vi "compare-trapezoid-profile-position-ctrl.vi"() -> ()   [LabVIEW 2019]
uses:
  Secret_Control_Library_Protected/CtrlTrain_Pos_ctrl_TuningParameters.ctl
  <vilib>/Rock Robotics/WPI/ThirdParty/JAS_Junk/TrajLib/SlewRateLimiter_New.vi
  <vilib>/Rock Robotics/WPI/ThirdParty/JAS_Junk/TrajLib/SlewRateLimiter_Reset.vi
  <vilib>/Rock Robotics/WPI/ThirdParty/JAS_Junk/TrajLib/SlewRateLimiter_Calculate.vi
  <vilib>/Rock Robotics/WPI/ThirdParty/JAS_Junk/TrajLib/SlewRateLimiter_SetRate.vi
  <vilib>/Rock Robotics/WPI/ThirdParty/JAS_Junk/TrajLib/TrapProfile_Calculate.vi
  <vilib>/Rock Robotics/WPI/ThirdParty/JAS_Junk/TrajLib/TrapProfile_New.vi
  <vilib>/Rock Robotics/WPI/ThirdParty/JAS_Junk/TrajLib/TrapProfile_TotalTime.vi
  <vilib>/Rock Robotics/WPI/ThirdParty/JAS_Junk/TrajLib/TrapProfConstraint_New.vi
  <vilib>/Rock Robotics/WPI/ThirdParty/JAS_Junk/TrajLib/TrapProfState_New.vi
  <vilib>/Rock Robotics/WPI/ThirdParty/JAS_Junk/TrajLib/TrapProfile_IsFinished.vi
  <vilib>/Rock Robotics/WPI/ThirdParty/JAS_Junk/TrajLib/TrapProfile_Direct.vi
  <vilib>/Rock Robotics/WPI/ThirdParty/JAS_Junk/TrajLib/TrapProfile_ShouldFlipAcceleration.vi
  <vilib>/Rock Robotics/SystemInterfaces/NetworkCommunication/NetComm_UsageReport_report.vi
  <vilib>/addons/control/pid/pid.llb/PID Lead-Lag (DBL).vi
  <vilib>/Rock Robotics/WPI/ThirdParty/JAS_Junk/TrajLib/Util_LibraryGlobals.vi
  <vilib>/Rock Robotics/WPI/ThirdParty/JAS_Junk/TrajLib/Util_GetTime.vi
  <vilib>/addons/control/pid/NI_PID_pid.lvlib
  <vilib>/Rock Robotics/WPI/ThirdParty/JAS_Junk/TrajLib/Trajectory_Library.lvlib
  Secret_Control_Library_Protected/Secret_Control_Library_Protected.lvlib
panel:
  in  "Tab Control":T1(tab)
  out "PC-SP, PV, CO Chart":T2(graph)
  in  "Desired Position":dbl(slide) min=0.0 max=90.0 scale=0.0..90.0
  in  "Auto - Set Position To 0 / Manual - Lower":bool
  in  "Auto - Set Position to 90 / Manual - Raise":bool
  in  "Set Position to Desired\n(Select to activate position)":bool
  out "Selected Setpoint \n(In Manual \ntracks Position)":dbl
  out "Trap-Current \nPosition 2":dbl format="%.2f"
  out "Trap-Motor \nDemand2":dbl format="%#.2f"
  out "Trap-Position Error":dbl format="%#3.2f"
  out "Trap-SP, PV, CO Chart":T2(graph)
  out "Trap-Current Position":dbl(knob) scale=-10.0..100.0
  in  "Auto / Manual":bool=TRUE
  in  "MinLimitSwitch":bool
  in  "MaxLimitSwitch":bool
  out "Trap-In Position":bool
  out "PC-Current \nPosition 2":dbl format="%.2f"
  out "PC-Motor \nDemand 2":dbl format="%#.2f"
  out "PC-Current Position 3":dbl(knob) scale=-10.0..100.0
  out "Selected Setpoint \n(In Manual \ntracks Position) 2":dbl
  out "PC-In Position":bool
  out "PC-Position Error":dbl format="%#3.2f"
  in  "MaxLimitSwitch 2":bool
  in  "MinLimitSwitch 2":bool
  in  "Trap-Max Accel":dbl=10.6 format="%#_13g"
  in  "PC-TuningParameters":T3={"MaxOutput"=1.0, "MinOutput"=0.25, "PositionErrThreshold"=6.0, "PositionErrDeadband"=0.5, "ReverseOutput"=FALSE, "PositionMax"=89.0, "PositionMin"=1.0, "WithinDBCount"=5} {"WithinDBCount" min=1}
  in  "trap-PositionTolerance":dbl=0.5 format="%#_13g"
  in  "Trap-VelocityTolerance":dbl=1.0 format="%#_13g"
  in  "Trap-ConsecutiveAtGoalCount":i32=5
  in  "Trap-Max Speed":dbl=8.5 format="%#_13g"
  in  "PC-MaxAccelRate":dbl=1.25 format="%#_13g"
  out "Both-Current-Setpoint":dbl
  out "Trap-Current-Position":dbl
  out "Both-Manual-Lower":bool
  out "Both-Manual-Raise":bool
  out "Trap-Motor-Demand":dbl
  out "PC-Current-Position":dbl
  out "PC-Motor-Demand":dbl
  # "Compare trapezoid with position control"
  # "Toggle these switches to simulate a limit switch input."
  # "Max Vel = 8.5"
  # "Max Output = 1.0"
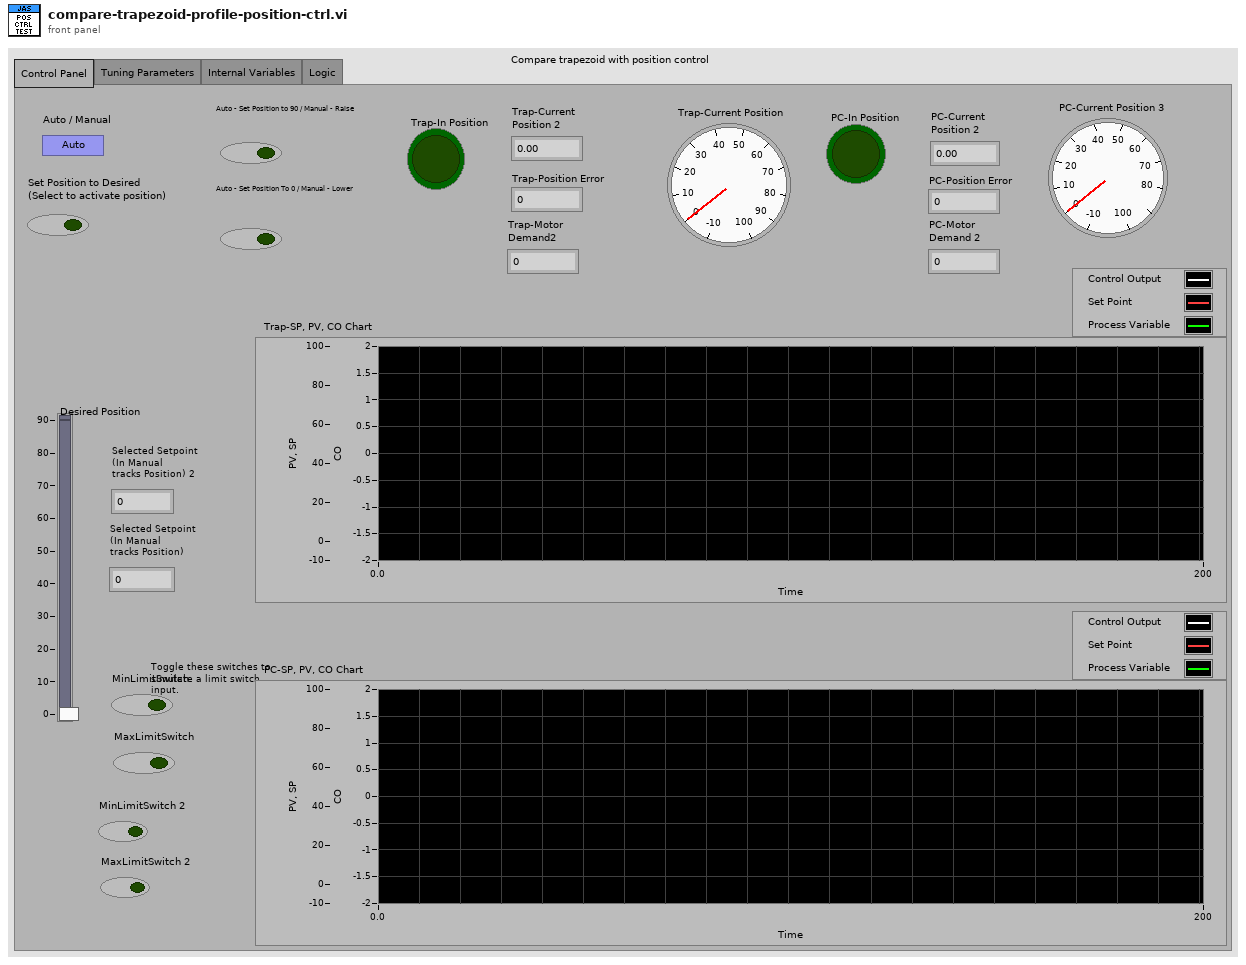
[diagram p1: front panel]
types:
  T1 = enum32{"Control Panel", "Tuning Parameters", "Internal Variables", "Logic"}
  T2 = cluster{"MotorDemand":dbl, "CurrentSetpoint":dbl, "CurrentPosition":dbl}
  T3 = typedef "Secret_Control_Library_Protected.lvlib/CtrlTrain_Pos_ctrl_TuningParameters.ctl" = cluster{"MaxOutput":dbl, "MinOutput":dbl, "PositionErrThreshold":dbl, "PositionErrDeadband":dbl, "ReverseOutput":bool, "PositionMax":dbl, "PositionMin":dbl, "WithinDBCount":i32}
  T4 = cluster{"gain":dbl, "lag time":dbl, "lead time":dbl}
  T5 = cluster{"PC-Motor-Demand":dbl, "Both-Current-Setpoint":dbl, "PC-Current-Position":dbl}
  T6 = cluster{"Trap-Motor-Demand":dbl, "Both-Current-Setpoint":dbl, "Trap-Current-Position":dbl}
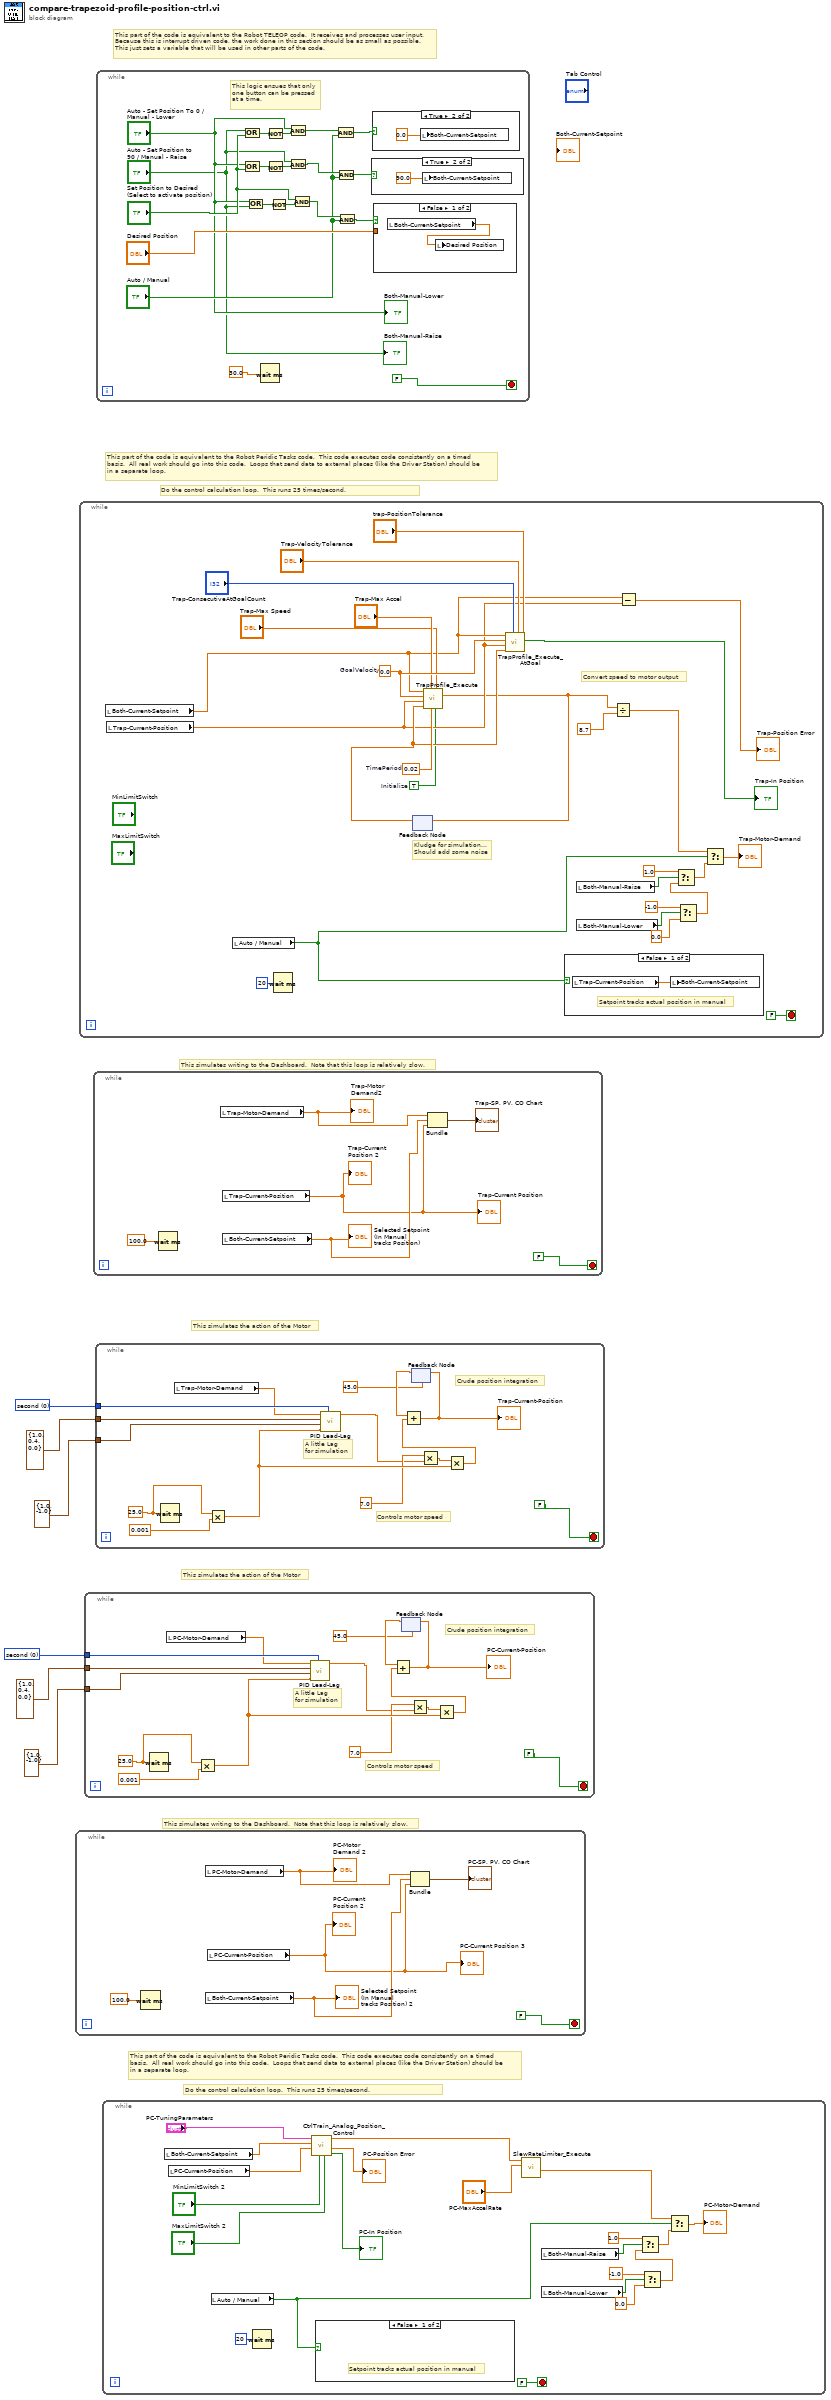
[diagram p0: block diagram]
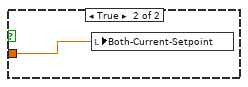
[diagram p4: hidden frame]
diagram:
  w1 = u16 0 items=["second", "minute"] ("time unit")
  w6 = u16 0 items=["second", "minute"] ("time unit")
  # "Do the control calculation loop.  This runs 25 times/second."
  # "This part of the code is equivalent to the Robot Peridic Tasks code.  This code executes code consistently on a timed\nbasis.  All real work should go into this code.  Loops that send data to external places (like the Driver Station) should be \nin a separate loop."
  # "This simulates writing to the Dashboard.  Note that this loop is relatively slow."
  # "This simulates the action of the Motor"
  # "This simulates the action of the Motor"
  # "This simulates writing to the Dashboard.  Note that this loop is relatively slow."
  # "Do the control calculation loop.  This runs 25 times/second."
  # "This part of the code is equivalent to the Robot Peridic Tasks code.  This code executes code consistently on a timed\nbasis.  All real work should go into this code.  Loops that send data to external places (like the Driver Station) should be \nin a separate loop."
  # "This part of the code is equivalent to the Robot TELEOP code.  It receives and processes user input.\nBecause this is interrupt driven code, the work done in this section should be as small as possible.\nThis just sets a variable that will be used in other parts of the code."
  n1 = while {
    stop <- FALSE stop-if-true
    n2 = Wait (ms)(milliseconds to wait=100.0) -> ()  [unwired: 1 out]
    n3 = local read "PC-Motor-Demand"() -> (w8:dbl)
    "PC-Motor \nDemand 2" <- w8
    n4 = local read "Both-Current-Setpoint"() -> (w10:dbl)
    "Selected Setpoint \n(In Manual \ntracks Position) 2" <- w10
    n5 = local read "PC-Current-Position"() -> (w9:dbl)
    "PC-Current \nPosition 2" <- w9
    "PC-Current Position 3" <- w9
    n6 = Bundle("PC-Motor-Demand"=w8, "Both-Current-Setpoint"=w10, "PC-Current-Position"=w9) -> (→"PC-SP, PV, CO Chart":T5)  [unwired: 1 in]
  }
  n7 = while {
    stop <- FALSE stop-if-true
    w29 = 0.0  # GoalVelocity
    w24 = 0.02  # TimePeriod
    w13 = TRUE  # Initialize
    # "Convert speed to motor output"
    # "Kludge for simulation...\nShould add some noise"
    n8 = local read "Both-Current-Setpoint"() -> (w21:dbl)
    n9 = local read "Trap-Current-Position"() -> (w17:dbl)
    n10 = local read "Auto / Manual"() -> (w34:bool)
    n11 = Wait (ms)(milliseconds to wait=u32 20) -> ()  [unwired: 1 out]
    n12 = feedback #1() -> (w18:dbl)  [unwired: 1 in]
    n13 = call <vilib>:"TrapProfile_Execute.vi"("Initialize"=w13, "Max Speed"="Trap-Max Speed", "TimePeriod"=w24, "Max Accel"="Trap-Max Accel", "CurrentVelocity"=w18, "CurrentPosition"=w17, "GoalVelocity"=w29, "GoalPosition"=w21) -> ("VelocityDmd"=w14:dbl)  [unwired: 3 out]
    n14 = feedback-in #1(w14) -> ()
    n15 = call <vilib>:"TrapProfile_Execute_AtGoal.vi"("PositionTolerance"="trap-PositionTolerance", "VelocityTolerance"="Trap-VelocityTolerance", "ConsecutiveAtGoalCount"="Trap-ConsecutiveAtGoalCount", "CurrentVelocity"=w18, "CurrentPosition"=w17, "GoalVelocity"=w29, "GoalPosition"=w21) -> ("AtGoal"=→"Trap-In Position":bool)  [unwired: 4 in]
    n16 = case shown="False" w34 {
      frame False {
        # "Setpoint tracks actual position in manual"
        n17 = local read "Trap-Current-Position"() -> (w40:dbl)
        n18 = local write "Both-Current-Setpoint"(w40) -> ()
      }
      frame True {
      }
    }
    n19 = local read "Both-Manual-Raise"() -> (w33:bool)
    n20 = local read "Both-Manual-Lower"() -> (w32:bool)
    n21 = Divide(x=w14, y=8.7) -> (x/y=w15:dbl)
    n22 = Subtract(x=w21, y=w17) -> (x-y=→"Trap-Position Error":dbl)
    n23 = Select(t=-1.0, s=w32, f=0.0) -> (s? t:f=w36:dbl)
    n24 = Select(t=1.0, s=w33, f=w36) -> (s? t:f=w35:dbl)
    n25 = Select(t=w15, s=w34, f=w35) -> (s? t:f=→"Trap-Motor-Demand":dbl)
  }
  n26 = while {
    tunnel: w1 -> [w55]
    tunnel: T4 {"gain"=1.0, "lag time"=0.4, "lead time"=0.0} ("tuning parameters") -> [w54]
    tunnel: cluster{"output high":dbl, "output low":dbl} {"output high"=1.0, "output low"=-1.0} ("output range") -> [w52]
    stop <- FALSE stop-if-true
    w44 = 25.0
    # "Controls motor speed"
    # "Crude position integration"
    # "A little Lag\nfor simulation"
    n27 = Wait (ms)(milliseconds to wait=w44) -> ()  [unwired: 1 out]
    n28 = local read "PC-Motor-Demand"() -> (w41:dbl)
    n29 = Multiply(x=w44, y=0.001) -> (x*y=w51:dbl)
    n30 = call-poly <vilib>:"PID Lead-Lag.vi"("time unit"=w55, "dt (s)"=w51, "output range"=w52, "tuning parameters"=w54, "input"=w41) -> ("output"=w43:dbl)  [unwired: 3 in, 1 out]
    n31 = feedback #2(45.0) -> (w49:dbl)
    n32 = Multiply(x=7.0, y=w43) -> (x*y=w50:dbl)
    n33 = Multiply(x=w50, y=w51) -> (x*y=w47:dbl)
    n34 = Add(x=w49, y=w47) -> (x+y=w42:dbl)
    "PC-Current-Position" <- w42
    n35 = feedback-in #2(w42) -> ()
  }
  n36 = while {
    stop <- FALSE stop-if-true
    n37 = Wait (ms)(milliseconds to wait=100.0) -> ()  [unwired: 1 out]
    n38 = local read "Trap-Motor-Demand"() -> (w56:dbl)
    "Trap-Motor \nDemand2" <- w56
    n39 = local read "Trap-Current-Position"() -> (w57:dbl)
    "Trap-Current \nPosition 2" <- w57
    "Trap-Current Position" <- w57
    n40 = local read "Both-Current-Setpoint"() -> (w58:dbl)
    "Selected Setpoint \n(In Manual \ntracks Position)" <- w58
    n41 = Bundle("Trap-Motor-Demand"=w56, "Both-Current-Setpoint"=w58, "Trap-Current-Position"=w57) -> (→"Trap-SP, PV, CO Chart":T6)  [unwired: 1 in]
  }
  n42 = while {
    tunnel: w6 -> [w76]
    tunnel: T4 {"gain"=1.0, "lag time"=0.4, "lead time"=0.0} ("tuning parameters") -> [w75]
    tunnel: cluster{"output high":dbl, "output low":dbl} {"output high"=1.0, "output low"=-1.0} ("output range") -> [w73]
    stop <- FALSE stop-if-true
    w65 = 25.0
    # "Controls motor speed"
    # "Crude position integration"
    # "A little Lag\nfor simulation"
    n43 = Wait (ms)(milliseconds to wait=w65) -> ()  [unwired: 1 out]
    n44 = local read "Trap-Motor-Demand"() -> (w62:dbl)
    n45 = Multiply(x=w65, y=0.001) -> (x*y=w72:dbl)
    n46 = call-poly <vilib>:"PID Lead-Lag.vi"("time unit"=w76, "dt (s)"=w72, "output range"=w73, "tuning parameters"=w75, "input"=w62) -> ("output"=w64:dbl)  [unwired: 3 in, 1 out]
    n47 = feedback #3(45.0) -> (w70:dbl)
    n48 = Multiply(x=7.0, y=w64) -> (x*y=w71:dbl)
    n49 = Multiply(x=w71, y=w72) -> (x*y=w68:dbl)
    n50 = Add(x=w70, y=w68) -> (x+y=w63:dbl)
    "Trap-Current-Position" <- w63
    n51 = feedback-in #3(w63) -> ()
  }
  n52 = while {
    stop <- FALSE stop-if-true
    # "This logic ensues that only\none button can be pressed\nat a time."
    n53 = Or(x="Auto - Set Position to 90 / Manual - Raise", y="Set Position to Desired\n(Select to activate position)") -> (x .or. y?=w95:bool)
    n54 = Or(x="Auto - Set Position To 0 / Manual - Lower", y="Set Position to Desired\n(Select to activate position)") -> (x .or. y?=w93:bool)
    n55 = Or(x="Auto - Set Position To 0 / Manual - Lower", y="Auto - Set Position to 90 / Manual - Raise") -> (x .or. y?=w91:bool)
    n56 = Wait (ms)(milliseconds to wait=30.0) -> ()  [unwired: 1 out]
    n57 = Not(x=w95) -> (.not. x?=w94:bool)
    n58 = Not(x=w93) -> (.not. x?=w92:bool)
    n59 = Not(x=w91) -> (.not. x?=w90:bool)
    n60 = And(x="Auto - Set Position To 0 / Manual - Lower", y=w94) -> (x .and. y?=w85:bool)
    n61 = And(x="Auto - Set Position to 90 / Manual - Raise", y=w92) -> (x .and. y?=w81:bool)
    n62 = And(x="Set Position to Desired\n(Select to activate position)", y=w90) -> (x .and. y?=w80:bool)
    n63 = And(x=w85, y="Auto / Manual") -> (x .and. y?=w84:bool)
    n64 = And(x=w81, y="Auto / Manual") -> (x .and. y?=w83:bool)
    n65 = And(x=w80, y="Auto / Manual") -> (x .and. y?=w82:bool)
    n66 = case shown="True" w83 {
      frame False {
      }
      frame True {
        n67 = local write "Both-Current-Setpoint"(90.0) -> ()
      }
    }
    n68 = case shown="True" w84 {
      frame False {
      }
      frame True {
        n69 = local write "Both-Current-Setpoint"(0.0) -> ()
      }
    }
    n70 = case shown="False" w82 {
      tunnel: "Desired Position" -> [_ w97]
      frame False {
        n71 = local read "Both-Current-Setpoint"() -> (w96:dbl)
        n72 = local write "Desired Position"(w96) -> ()
      }
      frame True {
        n73 = local write "Both-Current-Setpoint"(w97) -> ()
      }
    }
    "Both-Manual-Raise" <- "Auto - Set Position to 90 / Manual - Raise"
    "Both-Manual-Lower" <- "Auto - Set Position To 0 / Manual - Lower"
  }
  n74 = while {
    stop <- FALSE stop-if-true
    n75 = local read "Both-Current-Setpoint"() -> (w109:dbl)
    n76 = local read "PC-Current-Position"() -> (w108:dbl)
    n77 = local read "Auto / Manual"() -> (w115:bool)
    n78 = Wait (ms)(milliseconds to wait=u32 20) -> ()  [unwired: 1 out]
    n79 = call "CtrlTrain_Analog_Position_Control.vi"("PositionMax"="MaxLimitSwitch 2", "PositionMin"="MinLimitSwitch 2", "CurrentPosition"=w108, "TargetPosition"=w109, "Pos_Ctrl_TuningParameters"="PC-TuningParameters") -> ("OnTarget"=→"PC-In Position":bool, "PositionError"=→"PC-Position Error":dbl, "Output"=w101:dbl)  [unwired: 4 in]
    n80 = case shown="False" w115 {
      frame False {
        # "Setpoint tracks actual position in manual"
      }
      frame True {
      }
    }
    n81 = call <vilib>:"SlewRateLimiter_Execute.vi"("PositiveRate"="PC-MaxAccelRate", "Input"=w101) -> ("Output"=w100:dbl)  [unwired: 8 in, 1 out]
    n82 = local read "Both-Manual-Raise"() -> (w114:bool)
    n83 = local read "Both-Manual-Lower"() -> (w113:bool)
    n84 = Select(t=-1.0, s=w113, f=0.0) -> (s? t:f=w117:dbl)
    n85 = Select(t=1.0, s=w114, f=w117) -> (s? t:f=w116:dbl)
    n86 = Select(t=w100, s=w115, f=w116) -> (s? t:f=→"PC-Motor-Demand":dbl)
  }
